vi "子VI-工件信息输入.vi"(8 "Y Resolution":i32, 9 "X Resolution":i32) -> (0 "质量等级":string, 2 "框号字体大小-":i16, 3 "产品规格":cluster{"产品长度（周长）（mm）":dbl, "产品宽度（母线长）（mm）":dbl}, 4 "是否需要预处理":u16, 5 "图像分辨率":T1)   [LabVIEW 2018]
panel:
  in  "框号字体大小":i16
  in  "是否需要预处理（默认不进行预处理）":u16(ring) items=["需要预处理", "不需要预处理"]
  in  "质量等级（请填入A/B/C，默认为B）":u16(ring) items=["A", "B", "C"]
  out "错误常量out":errorcluster
  in  "错误常量":errorcluster
  in  "停止按钮":bool
  in  "产品宽度（母线长）（mm）":dbl format="%#_13g"
  in  "产品长度（周长）（mm）":dbl format="%#_13g"
  in  "长度方向分辨率（Y方向-mm/像素）":dbl=1.0 format="%#_13g"
  in  "宽度方向分辨率（X方向-mm/像素）":dbl=1.0 format="%#_13g"
  # "图像及工件参数输入"
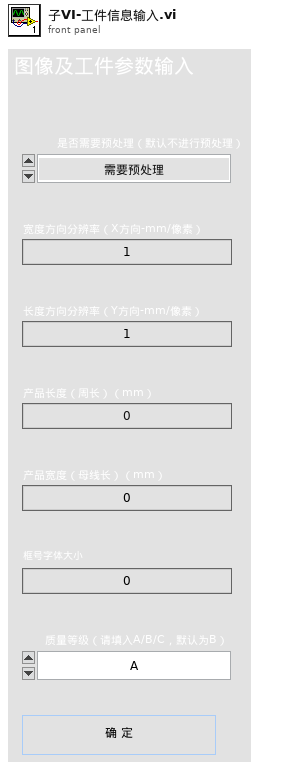
[diagram p1: front panel]
types:
  T1 = cluster{"图像X向分辨率（mm/像素）":dbl, "图像Y向分辨率（mm/像素）":dbl}
  T2 = cluster{"宽度方向分辨率（X方向-mm/像素）":dbl, "长度方向分辨率（Y方向-mm/像素）":dbl}
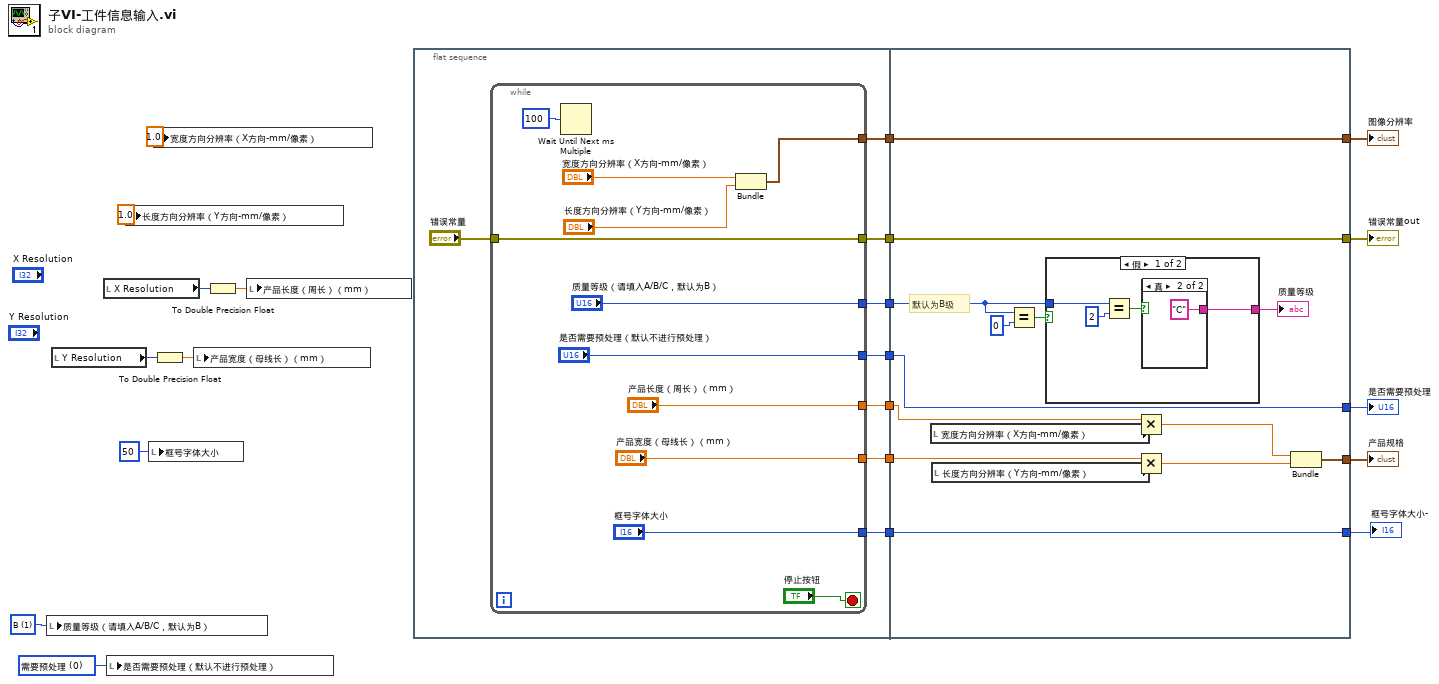
[diagram p0: block diagram]
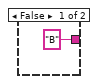
[diagram p2: hidden frame]
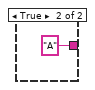
[diagram p3: hidden frame]
diagram:
  w11 = u16 0 items=["需要预处理", "不需要预处理"] ("是否需要预处理（默认不进行预处理）")
  w18 = u16 1 items=["A", "B", "C"] ("质量等级（请填入A/B/C，默认为B）")
  n1 = local write "质量等级（请填入A/B/C，默认为B）"(w18) -> ()
  n2 = local read "Y Resolution"() -> (w15:i32)
  n3 = local read "X Resolution"() -> (w17:i32)
  n4 = local write "是否需要预处理（默认不进行预处理）"(w11) -> ()
  n5 = local write "长度方向分辨率（Y方向-mm/像素）"(1.0 ("图像Y向分辨率（mm/像素）")) -> ()
  n6 = local write "框号字体大小"(i8 50 ("框号字体大小")) -> ()
  n7 = local write "宽度方向分辨率（X方向-mm/像素）"(1.0 ("图像X向分辨率（mm/像素）")) -> ()
  n8 = To Double Precision Float(number=w15) -> (double precision float=w14:dbl)
  n9 = local write "产品宽度（母线长）（mm）"(w14) -> ()
  n10 = To Double Precision Float(number=w17) -> (double precision float=w16:dbl)
  n11 = local write "产品长度（周长）（mm）"(w16) -> ()
  n12 = flat-sequence {
    tunnel: [w29] -> w10
    tunnel: [w28] -> w9
    tunnel: [w27] -> w8
    tunnel: [w25] -> w7
    tunnel: [w24] -> w5
    tunnel: [w23] -> w4
    tunnel: [w22] -> w2
    tunnel: [w54] -> w19
    tunnel: [w48] -> w20
    tunnel: [w55] -> w21
    tunnel: w10 -> [w55]
    tunnel: w9 -> [w54]
    tunnel: w8 -> [w51]
    tunnel: w7 -> [w49]
    tunnel: [w49] -> w6
    tunnel: w5 -> [w47]
    tunnel: w4 -> [w43]
    tunnel: [w41] -> w1
    tunnel: w2 -> [w41]
    frame #0 {
      n13 = while {
        tunnel: [w40] -> w29
        tunnel: "错误常量" -> [w36]
        tunnel: [w36] -> w28
        tunnel: ["质量等级（请填入A/B/C，默认为B）"] -> w27
        tunnel: ["是否需要预处理（默认不进行预处理）"] -> w25
        tunnel: ["产品长度（周长）（mm）"] -> w24
        tunnel: ["产品宽度（母线长）（mm）"] -> w23
        tunnel: ["框号字体大小"] -> w22
        stop <- "停止按钮" stop-if-true
        n14 = Wait Until Next ms Multiple(millisecond multiple=u32 100 ("毫秒倍数")) -> ()  [unwired: 1 out]
        n15 = Bundle("宽度方向分辨率（X方向-mm/像素）"="宽度方向分辨率（X方向-mm/像素）", "长度方向分辨率（Y方向-mm/像素）"="长度方向分辨率（Y方向-mm/像素）") -> (w40:T2)  [unwired: 1 in]
      }
    }
    frame #1 {
      # "默认为B级"
      n16 = local read "宽度方向分辨率（X方向-mm/像素）"() -> (w46:dbl)
      n17 = local read "长度方向分辨率（Y方向-mm/像素）"() -> (w42:dbl)
      n18 = Equal?(x=w51, y=u16 0) -> (x = y?=w52:bool)
      n19 = case shown="假" w52 {
        tunnel: [w56 "A" ("质量等级")] -> w53
        tunnel: w51 -> [w58 _]
        frame False {
          n20 = Equal?(x=w58, y=u16 2) -> (x = y?=w57:bool)
          n21 = case shown="真" w57 {
            tunnel: ["B" ("质量等级") "C" ("质量等级")] -> w56
            frame False {
            }
            frame True {
            }
          }
        }
        frame True {
        }
      }
      "质量等级" <- w53
      n22 = Multiply(x=w47, y=w46) -> (x*y=w45:dbl)
      n23 = Multiply(x=w43, y=w42) -> (x*y=w44:dbl)
      n24 = Bundle(w45, w44) -> (w48:cluster{dbl, dbl})  [unwired: 1 in]
    }
  }
  "图像分辨率" <- w21
  "产品规格" <- w20
  "错误常量out" <- w19
  "是否需要预处理" <- w6
  "框号字体大小-" <- w1
